vi "Configure Level Settings.vi"(0 "VISA resource name":refnum<visa-resource-name>, 1 "Level Offset State (0:Off)":i32(ring) items=["Off", "On", "Set Level"], 2 "Level Offset (0.00dB)":dbl min=-100.0 max=100.0 format="%.2f", 3 "Reference Level (-10.00dBm)":dbl=-10.0 min=-120.0 max=50.0 format="%.2f", 5 "Attenuator (10.00dB)":i32=10 min=0 max=60 format="%.2f", 7 "Auto  Attenuator(0:Auto)":i32(ring) items=["Auto", "1 Step Up", "1 Step Down", "Set Attenuator Value"], 9 "Attenuator Step (0:2dB)":i32(ring) items=["2dB", "10dB"], 11 "error in (no error)":errorcluster, 14 "Enable Offset (F:Disable)":bool) -> (4 "VISA resource name out":refnum<visa-resource-name>, 15 "error out":errorcluster)   [LabVIEW 2023, in "Anritsu Signal Analyzer Series.lvlib"]
doc: "Configures the vertical settings of the spectrum analyzer."
uses:
  Anritsu Signal Analyzer Series.lvlib
panel:
  # "dB"
  # "dB"
  # "dBm"
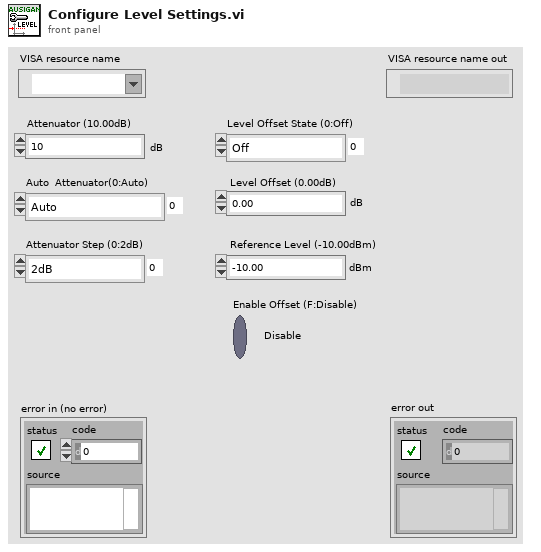
[diagram p1: front panel]
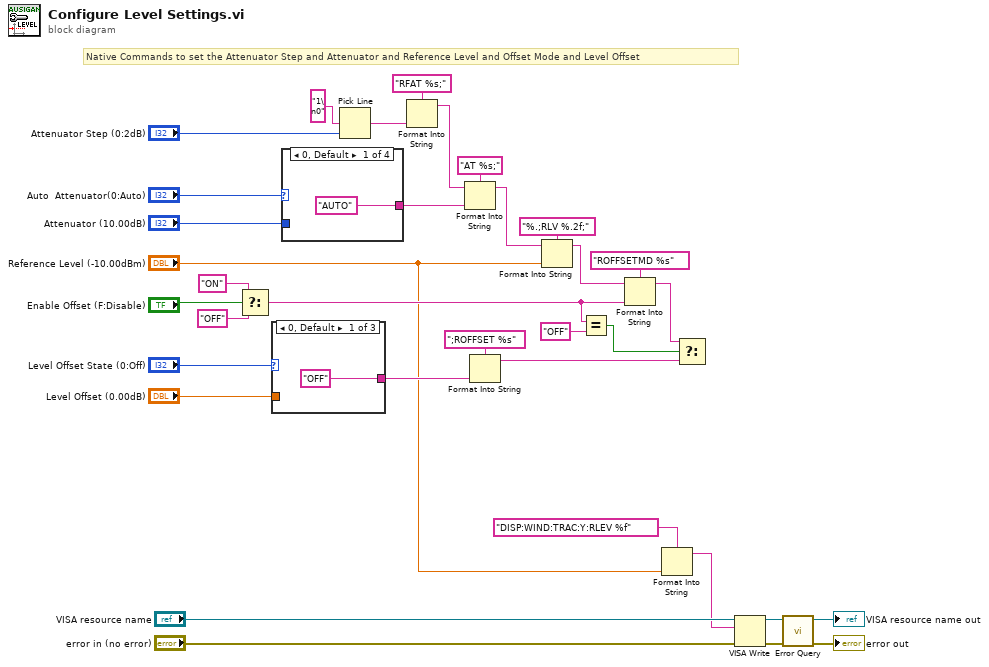
[diagram p0: block diagram]
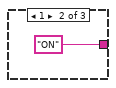
[diagram p2: hidden frame]
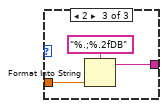
[diagram p3: hidden frame]
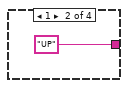
[diagram p4: hidden frame]
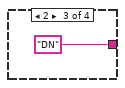
[diagram p5: hidden frame]
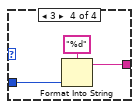
[diagram p6: hidden frame]
diagram:
  # "Native Commands to set the Attenuator Step and Attenuator and Reference Level and Offset Mode and Level Offset"
  n1 = Select(t="ON", s="Enable Offset (F:Disable)", f="OFF") -> (s? t:f=w7:string)
  n2 = case shown="0, Default" "Level Offset State (0:Off)" {
    tunnel: ["OFF" ("_Case0") "ON" ("_Case1") w38] -> w15
    tunnel: "Level Offset (0.00dB)" -> [_ _ w37]
    frame 0, Default {
    }
    frame 1 {
    }
    frame 2 {
      n3 = Format Into String(format string="%.;%.2fDB", w37) -> (resulting string=w38:string)  [unwired: 2 in, 1 out]
    }
  }
  n4 = case shown="0, Default" "Auto  Attenuator(0:Auto)" {
    tunnel: ["AUTO" "UP" "DN" w44] -> w18
    tunnel: "Attenuator (10.00dB)" -> [_ _ _ w43]
    frame 0, Default {
    }
    frame 1 {
    }
    frame 2 {
    }
    frame 3 {
      n5 = Format Into String(format string="%d", w43) -> (resulting string=w44:string)  [unwired: 2 in, 1 out]
    }
  }
  n6 = Pick Line(multi-line string="1\n0" ("複数行文字列"), line index="Attenuator Step (0:2dB)") -> (output string=w23:string)  [unwired: 1 in]
  n7 = Format Into String(format string="RFAT %s;" ("_CommandSet"), w23) -> (resulting string=w17:string)  [unwired: 2 in, 1 out]
  n8 = Format Into String(format string="AT %s;" ("_CommandSet"), initial string=w17, w18) -> (resulting string=w16:string)  [unwired: 1 in, 1 out]
  n9 = Format Into String(format string=";ROFFSET %s" ("_CommandSet"), w15) -> (resulting string=w6:string)  [unwired: 2 in, 1 out]
  n10 = Format Into String(format string="%.;RLV %.2f;" ("Format String"), initial string=w16, "Reference Level (-10.00dBm)") -> (resulting string=w21:string)  [unwired: 1 in, 1 out]
  n11 = Equal?(x=w7, y="OFF") -> (x = y?=w4:bool)
  n12 = Format Into String(format string="ROFFSETMD %s" ("_CommandSet"), initial string=w21, w7) -> (resulting string=w5:string)  [unwired: 1 in, 1 out]
  n13 = Format Into String(format string="DISP:WIND:TRAC:Y:RLEV %f", "Reference Level (-10.00dBm)") -> (resulting string=w2:string)  [unwired: 2 in, 1 out]
  n14 = Select(t=w5, s=w4, f=w6) -> ()  [unwired: 1 out]
  n15 = VISA Write(VISA resource name="VISA resource name", write buffer=w2, error in (no error)="error in (no error)") -> (VISA resource name out=w12:refnum<visa-resource-name>, error out=w11:errorcluster)  [unwired: 1 out]
  n16 = call "Error Query.vi"("error in (no error)"=w11, "VISA resource name"=w12) -> ("error out"=→"error out":errorcluster, "VISA resource name out"=→"VISA resource name out":refnum<visa-resource-name>)  [unwired: 6 in, 2 out]
